vi "bitpacking_acquire_push.vi"(8 "sample":i16, 9 "Debug":bool=TRUE, 10 "Input Valid":bool, 11 "FIFO Refs":T1={"FIFO 0"="Simulation FIFO 0", "FIFO 1"="Simulation FIFO 1", "FIFO 2"="Simulation FIFO 2", "FIFO 3"="Simulation FIFO 3", "FIFO 4"="Simulation FIFO 4", "FIFO 5"="Simulation FIFO 5"}) -> (3 "Ready for Input":bool)   [LabVIEW 2014]
uses:
  FPGA_Controls/Acquisition FIFOs Cluster.ctl
  <vilib>/rvi/eio/common/nirviEmuTemplateMethod_errors.vi
  <vilib>/rvi/DataTransferAndStorage/Container/Common/niFpgaContainerExecOnDevCompGetState.vi
  <vilib>/rvi/Emulation/niFpgaEmulationIsFPGAContextNoSignature.vi
  <vilib>/rvi/Emulation/niFpgaSctlEmulationGetInTimedLoop.vi
  <vilib>/rvi/errors/niFpgaSetErrorForExecOnDevCompSimple.vi
  <vilib>/rvi/eio/common/nirviEmuReportErrorAndStop.vi
  <vilib>/rvi/DataTransferAndStorage/Container/Common/niFpgaContainerGetUniqueNameForEmu.vi
  <vilib>/rvi/FIFO/Fifo_Resource/nirvififoEmulationSetSize.vi
  <vilib>/rvi/FIFO/Fifo_Resource/nirviFifoEmulationQueueMgr.vi
  <instcachedir>/0/nirviFifoEmulationQueueMgr_E5CAEC123FF24DC58D834DCA3CDAA9B5.lvgen/nirviFifoEmulationQueueMgr_E5CAEC123FF24DC58D834DCA3CDAA9B5_003.vi
  <vilib>/rvi/FIFO/Fifo_Resource/nirvififoEmulationDetermineInputValidOut.vi
  <vilib>/rvi/FIFO/Fifo_Resource/nirvififoEmulationCreateLock.vi
  <vilib>/rvi/Emulation/niFpgaProcessEmulError.vi
  <vilib>/rvi/FIFO/Fifo_Resource/nirvififoEmulationObtainLock.vi
  <vilib>/rvi/FIFO/Fifo_Resource/nirvififoEmulationReleaseLock.vi
  <vilib>/rvi/occurrence/nirviWaitOnOccurrenceBase.vi
  <vilib>/rvi/errors/nirviReportUnexpectedCaseInternalError.vi
  <vilib>/rvi/errors/nirviReportUnexpectedCaseInternalError (U32).vi
  <vilib>/Utility/error.llb/Clear Errors.vi
  <vilib>/rvi/interface/RandomDataEmulation/niFpgaRandomDataHandleErrors.vi
  <vilib>/eio/EIONode/EIONode.xnode
  <vilib>/rvi/DataTransferAndStorage/Container/XNode/niFpgaContainer.xnode
  <vilib>/rvi/FIFO/Fifo_Resource/niFpgaFifoEmulationRefIn.vi
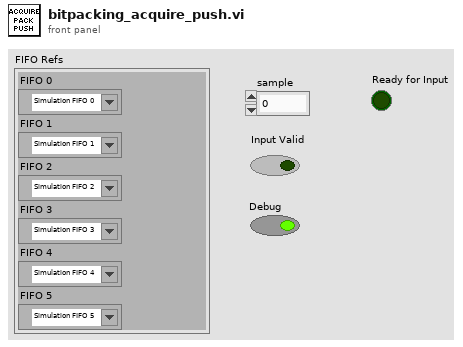
[diagram p1: front panel]
types:
  T1 = typedef "Acquisition FIFOs Cluster.ctl" = cluster{"FIFO 0":refnum<k21>, "FIFO 1":refnum<k21>, "FIFO 2":refnum<k21>, "FIFO 3":refnum<k21>, "FIFO 4":refnum<k21>, "FIFO 5":refnum<k21>}
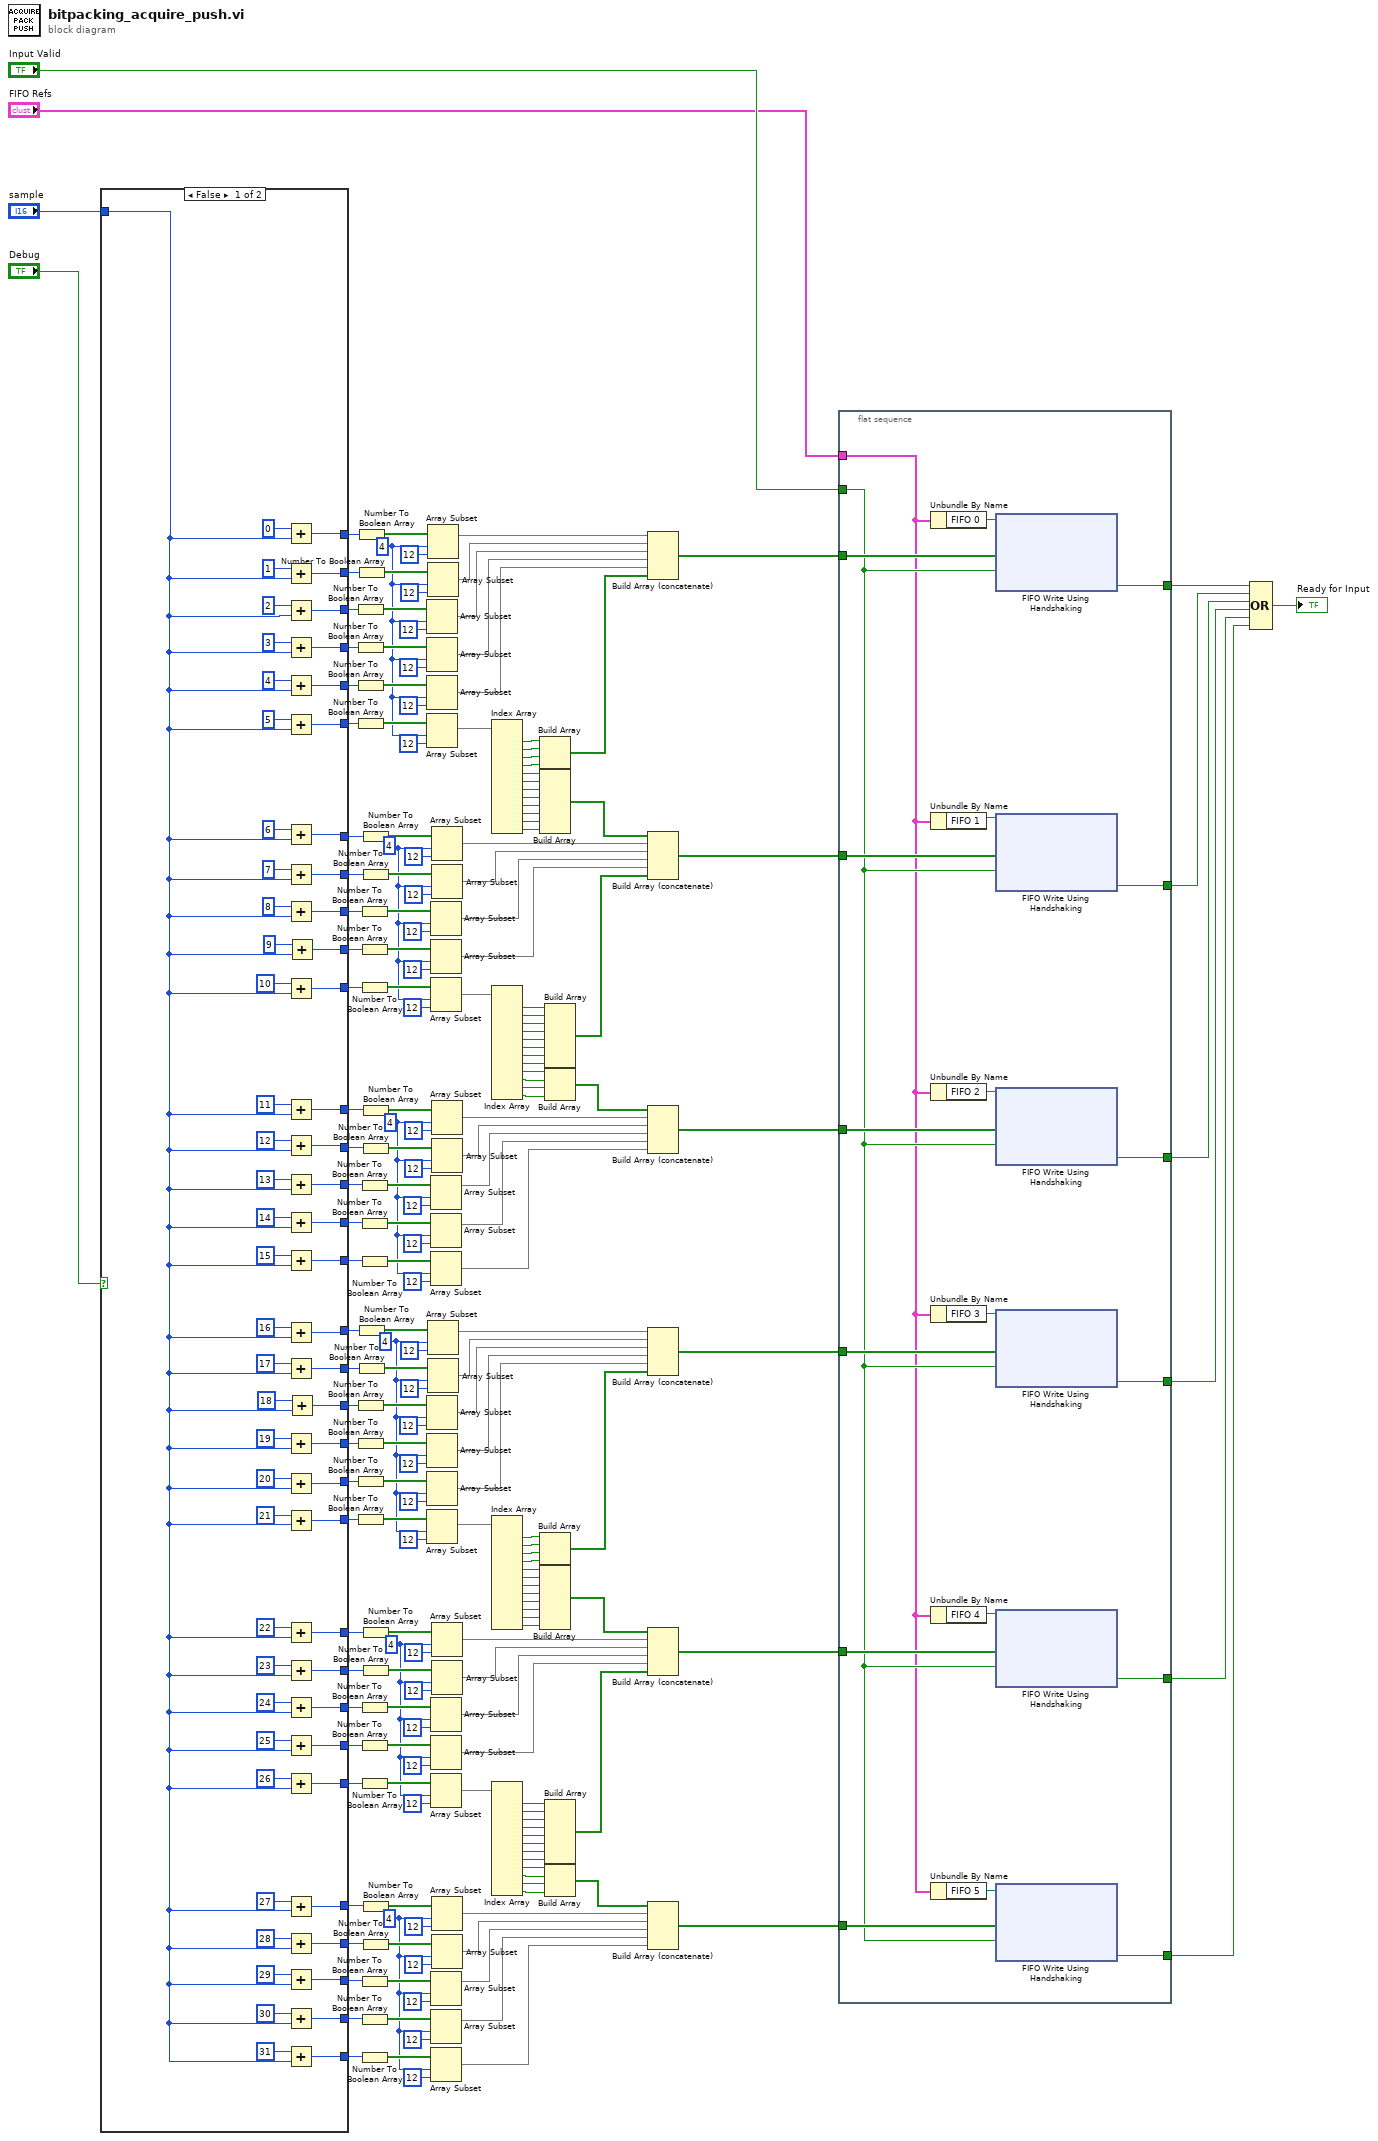
[diagram p0: block diagram]
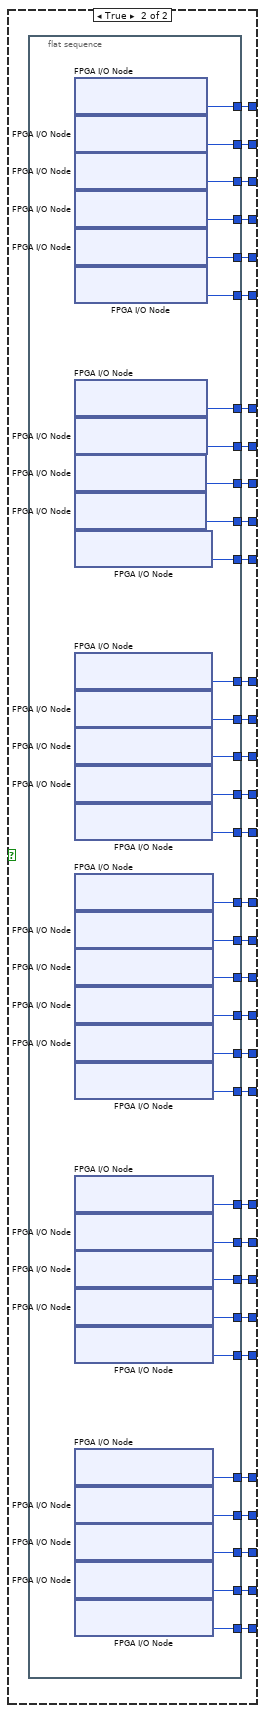
[diagram p2: hidden frame]
diagram:
  w3 = 4 ("length")
  w4 = 4 ("index")
  w5 = 4 ("index")
  w6 = 4 ("index")
  w7 = 4 ("index")
  w8 = 4 ("index")
  n1 = case shown="False" "Debug" {
    tunnel: [w219 w304] -> w125
    tunnel: [w218 w303] -> w124
    tunnel: [w217 w302] -> w123
    tunnel: [w216 w301] -> w122
    tunnel: [w215 w300] -> w121
    tunnel: [w214 w299] -> w120
    tunnel: [w213 w298] -> w119
    tunnel: [w212 w297] -> w118
    tunnel: [w211 w296] -> w117
    tunnel: [w210 w295] -> w116
    tunnel: [w209 w294] -> w115
    tunnel: [w240 w293] -> w114
    tunnel: [w239 w292] -> w113
    tunnel: [w238 w291] -> w112
    tunnel: [w237 w290] -> w111
    tunnel: [w236 w289] -> w110
    tunnel: [w220 w288] -> w103
    tunnel: [w221 w287] -> w102
    tunnel: [w222 w286] -> w101
    tunnel: [w223 w285] -> w100
    tunnel: [w224 w284] -> w99
    tunnel: [w225 w283] -> w98
    tunnel: [w226 w282] -> w97
    tunnel: [w227 w281] -> w96
    tunnel: [w228 w280] -> w95
    tunnel: [w229 w279] -> w94
    tunnel: [w230 w278] -> w93
    tunnel: [w231 w277] -> w92
    tunnel: [w232 w276] -> w91
    tunnel: [w233 w275] -> w90
    tunnel: [w234 w274] -> w89
    tunnel: [w235 w273] -> w88
    tunnel: "sample" -> [w208 _]
    frame False {
      n2 = Add(x=i16 0, y=w208) -> (x+y=w235:i16)
      n3 = Add(x=i16 1, y=w208) -> (x+y=w234:i16)
      n4 = Add(x=i16 2, y=w208) -> (x+y=w233:i16)
      n5 = Add(x=i16 3, y=w208) -> (x+y=w232:i16)
      n6 = Add(x=i16 4, y=w208) -> (x+y=w231:i16)
      n7 = Add(x=i16 5, y=w208) -> (x+y=w230:i16)
      n8 = Add(x=i16 6, y=w208) -> (x+y=w229:i16)
      n9 = Add(x=i16 7, y=w208) -> (x+y=w228:i16)
      n10 = Add(x=i16 8, y=w208) -> (x+y=w227:i16)
      n11 = Add(x=i16 10, y=w208) -> (x+y=w225:i16)
      n12 = Add(x=i16 11, y=w208) -> (x+y=w224:i16)
      n13 = Add(x=i16 12, y=w208) -> (x+y=w223:i16)
      n14 = Add(x=i16 13, y=w208) -> (x+y=w222:i16)
      n15 = Add(x=i16 14, y=w208) -> (x+y=w221:i16)
      n16 = Add(x=i16 15, y=w208) -> (x+y=w220:i16)
      n17 = Add(x=i16 16, y=w208) -> (x+y=w219:i16)
      n18 = Add(x=i16 17, y=w208) -> (x+y=w218:i16)
      n19 = Add(x=i16 19, y=w208) -> (x+y=w216:i16)
      n20 = Add(x=i16 20, y=w208) -> (x+y=w215:i16)
      n21 = Add(x=i16 21, y=w208) -> (x+y=w214:i16)
      n22 = Add(x=i16 22, y=w208) -> (x+y=w213:i16)
      n23 = Add(x=i16 23, y=w208) -> (x+y=w212:i16)
      n24 = Add(x=i16 24, y=w208) -> (x+y=w211:i16)
      n25 = Add(x=i16 25, y=w208) -> (x+y=w210:i16)
      n26 = Add(x=i16 26, y=w208) -> (x+y=w209:i16)
      n27 = Add(x=i16 27, y=w208) -> (x+y=w240:i16)
      n28 = Add(x=i16 28, y=w208) -> (x+y=w239:i16)
      n29 = Add(x=i16 29, y=w208) -> (x+y=w238:i16)
      n30 = Add(x=i16 30, y=w208) -> (x+y=w237:i16)
      n31 = Add(x=i16 31, y=w208) -> (x+y=w236:i16)
      n32 = Add(x=i16 9, y=w208) -> (x+y=w226:i16)
      n33 = Add(x=i16 18, y=w208) -> (x+y=w217:i16)
    }
    frame True {
      n34 = flat-sequence {
        tunnel: [w336] -> w273
        tunnel: [w335] -> w274
        tunnel: [w334] -> w275
        tunnel: [w333] -> w276
        tunnel: [w332] -> w277
        tunnel: [w331] -> w278
        tunnel: [w330] -> w279
        tunnel: [w329] -> w280
        tunnel: [w328] -> w281
        tunnel: [w327] -> w282
        tunnel: [w326] -> w283
        tunnel: [w325] -> w284
        tunnel: [w324] -> w285
        tunnel: [w323] -> w286
        tunnel: [w322] -> w287
        tunnel: [w321] -> w288
        tunnel: [w320] -> w289
        tunnel: [w319] -> w290
        tunnel: [w318] -> w291
        tunnel: [w317] -> w292
        tunnel: [w316] -> w293
        tunnel: [w315] -> w294
        tunnel: [w314] -> w295
        tunnel: [w313] -> w296
        tunnel: [w312] -> w297
        tunnel: [w311] -> w298
        tunnel: [w310] -> w299
        tunnel: [w309] -> w300
        tunnel: [w308] -> w301
        tunnel: [w307] -> w302
        tunnel: [w306] -> w303
        tunnel: [w305] -> w304
        frame #0 {
          n35 = xnode "FPGA I/O Node"() -> ("IO Module\\AI A0"=w336:i16)  [unwired: 1 in, 1 out]
          n36 = xnode "FPGA I/O Node"() -> ("IO Module\\AI A1"=w335:i16)  [unwired: 1 in, 1 out]
          n37 = xnode "FPGA I/O Node"() -> ("IO Module\\AI A2"=w334:i16)  [unwired: 1 in, 1 out]
          n38 = xnode "FPGA I/O Node"() -> ("IO Module\\AI A3"=w333:i16)  [unwired: 1 in, 1 out]
          n39 = xnode "FPGA I/O Node"() -> ("IO Module\\AI A4"=w332:i16)  [unwired: 1 in, 1 out]
          n40 = xnode "FPGA I/O Node"() -> ("IO Module\\AI A5"=w331:i16)  [unwired: 1 in, 1 out]
          n41 = xnode "FPGA I/O Node"() -> ("IO Module\\AI A6"=w330:i16)  [unwired: 1 in, 1 out]
          n42 = xnode "FPGA I/O Node"() -> ("IO Module\\AI A7"=w329:i16)  [unwired: 1 in, 1 out]
          n43 = xnode "FPGA I/O Node"() -> ("IO Module\\AI B8"=w328:i16)  [unwired: 1 in, 1 out]
          n44 = xnode "FPGA I/O Node"() -> ("IO Module\\AI B9"=w327:i16)  [unwired: 1 in, 1 out]
          n45 = xnode "FPGA I/O Node"() -> ("IO Module\\AI B10"=w326:i16)  [unwired: 1 in, 1 out]
          n46 = xnode "FPGA I/O Node"() -> ("IO Module\\AI B11"=w325:i16)  [unwired: 1 in, 1 out]
          n47 = xnode "FPGA I/O Node"() -> ("IO Module\\AI B12"=w324:i16)  [unwired: 1 in, 1 out]
          n48 = xnode "FPGA I/O Node"() -> ("IO Module\\AI B13"=w323:i16)  [unwired: 1 in, 1 out]
          n49 = xnode "FPGA I/O Node"() -> ("IO Module\\AI B14"=w322:i16)  [unwired: 1 in, 1 out]
          n50 = xnode "FPGA I/O Node"() -> ("IO Module\\AI B15"=w321:i16)  [unwired: 1 in, 1 out]
          n51 = xnode "FPGA I/O Node"() -> ("IO Module\\AI C16"=w305:i16)  [unwired: 1 in, 1 out]
          n52 = xnode "FPGA I/O Node"() -> ("IO Module\\AI C17"=w306:i16)  [unwired: 1 in, 1 out]
          n53 = xnode "FPGA I/O Node"() -> ("IO Module\\AI C18"=w307:i16)  [unwired: 1 in, 1 out]
          n54 = xnode "FPGA I/O Node"() -> ("IO Module\\AI C19"=w308:i16)  [unwired: 1 in, 1 out]
          n55 = xnode "FPGA I/O Node"() -> ("IO Module\\AI C20"=w309:i16)  [unwired: 1 in, 1 out]
          n56 = xnode "FPGA I/O Node"() -> ("IO Module\\AI C21"=w310:i16)  [unwired: 1 in, 1 out]
          n57 = xnode "FPGA I/O Node"() -> ("IO Module\\AI C22"=w311:i16)  [unwired: 1 in, 1 out]
          n58 = xnode "FPGA I/O Node"() -> ("IO Module\\AI C23"=w312:i16)  [unwired: 1 in, 1 out]
          n59 = xnode "FPGA I/O Node"() -> ("IO Module\\AI D24"=w313:i16)  [unwired: 1 in, 1 out]
          n60 = xnode "FPGA I/O Node"() -> ("IO Module\\AI D25"=w314:i16)  [unwired: 1 in, 1 out]
          n61 = xnode "FPGA I/O Node"() -> ("IO Module\\AI D26"=w315:i16)  [unwired: 1 in, 1 out]
          n62 = xnode "FPGA I/O Node"() -> ("IO Module\\AI D27"=w316:i16)  [unwired: 1 in, 1 out]
          n63 = xnode "FPGA I/O Node"() -> ("IO Module\\AI D28"=w317:i16)  [unwired: 1 in, 1 out]
          n64 = xnode "FPGA I/O Node"() -> ("IO Module\\AI D29"=w318:i16)  [unwired: 1 in, 1 out]
          n65 = xnode "FPGA I/O Node"() -> ("IO Module\\AI D30"=w319:i16)  [unwired: 1 in, 1 out]
          n66 = xnode "FPGA I/O Node"() -> ("IO Module\\AI D31"=w320:i16)  [unwired: 1 in, 1 out]
        }
      }
    }
  }
  n67 = Number To Boolean Array(number=w90) -> (Boolean array=w21:bool[])
  n68 = Number To Boolean Array(number=w91) -> (Boolean array=w18:bool[])
  n69 = Number To Boolean Array(number=w92) -> (Boolean array=w27:bool[])
  n70 = Number To Boolean Array(number=w93) -> (Boolean array=w24:bool[])
  n71 = Number To Boolean Array(number=w123) -> (Boolean array=w192:bool[])
  n72 = Number To Boolean Array(number=w122) -> (Boolean array=w195:bool[])
  n73 = Number To Boolean Array(number=w121) -> (Boolean array=w186:bool[])
  n74 = Number To Boolean Array(number=w120) -> (Boolean array=w189:bool[])
  n75 = Number To Boolean Array(number=w88) -> (Boolean array=w12:bool[])
  n76 = Number To Boolean Array(number=w89) -> (Boolean array=w15:bool[])
  n77 = Number To Boolean Array(number=w125) -> (Boolean array=w201:bool[])
  n78 = Number To Boolean Array(number=w124) -> (Boolean array=w198:bool[])
  n79 = Number To Boolean Array(number=w96) -> (Boolean array=w45:bool[])
  n80 = Number To Boolean Array(number=w97) -> (Boolean array=w48:bool[])
  n81 = Number To Boolean Array(number=w98) -> (Boolean array=w43:bool[])
  n82 = Number To Boolean Array(number=w101) -> (Boolean array=w79:bool[])
  n83 = Number To Boolean Array(number=w102) -> (Boolean array=w76:bool[])
  n84 = Number To Boolean Array(number=w103) -> (Boolean array=w81:bool[])
  n85 = Number To Boolean Array(number=w117) -> (Boolean array=w168:bool[])
  n86 = Number To Boolean Array(number=w116) -> (Boolean array=w165:bool[])
  n87 = Number To Boolean Array(number=w115) -> (Boolean array=w170:bool[])
  n88 = Number To Boolean Array(number=w112) -> (Boolean array=w134:bool[])
  n89 = Number To Boolean Array(number=w111) -> (Boolean array=w137:bool[])
  n90 = Number To Boolean Array(number=w110) -> (Boolean array=w132:bool[])
  n91 = Number To Boolean Array(number=w94) -> (Boolean array=w52:bool[])
  n92 = Number To Boolean Array(number=w95) -> (Boolean array=w49:bool[])
  n93 = Number To Boolean Array(number=w99) -> (Boolean array=w72:bool[])
  n94 = Number To Boolean Array(number=w100) -> (Boolean array=w75:bool[])
  n95 = Number To Boolean Array(number=w119) -> (Boolean array=w161:bool[])
  n96 = Number To Boolean Array(number=w118) -> (Boolean array=w164:bool[])
  n97 = Number To Boolean Array(number=w114) -> (Boolean array=w141:bool[])
  n98 = Number To Boolean Array(number=w113) -> (Boolean array=w138:bool[])
  n99 = Array Subset(array=w21, index=w8, length=12) -> (w22:bool[])
  n100 = Array Subset(array=w18, index=w8, length=12) -> (w23:bool[])
  n101 = Array Subset(array=w27, index=w8, length=12) -> (w28:bool[])
  n102 = Array Subset(array=w24, index=w8, length=12) -> (w29:bool[])
  n103 = Array Subset(array=w192, index=w5, length=12) -> (w191:bool[])
  n104 = Array Subset(array=w195, index=w5, length=12) -> (w190:bool[])
  n105 = Array Subset(array=w186, index=w5, length=12) -> (w185:bool[])
  n106 = Array Subset(array=w189, index=w5, length=12) -> (w184:bool[])
  n107 = Array Subset(array=w12, index=w8, length=12) -> (w16:bool[])
  n108 = Array Subset(array=w15, index=w8, length=12) -> (w17:bool[])
  n109 = Array Subset(array=w201, index=w5, length=12) -> (w197:bool[])
  n110 = Array Subset(array=w198, index=w5, length=12) -> (w196:bool[])
  n111 = Array Subset(array=w45, index=w7, length=12) -> (w56:bool[])
  n112 = Array Subset(array=w48, index=w7, length=12) -> (w57:bool[])
  n113 = Array Subset(array=w43, index=w7, length=12) -> (w58:bool[])
  n114 = Array Subset(array=w79, index=w6, length=12) -> (w85:bool[])
  n115 = Array Subset(array=w76, index=w6, length=12) -> (w86:bool[])
  n116 = Array Subset(array=w81, index=w6, length=12) -> (w87:bool[])
  n117 = Array Subset(array=w168, index=w4, length=12) -> (w157:bool[])
  n118 = Array Subset(array=w165, index=w4, length=12) -> (w156:bool[])
  n119 = Array Subset(array=w170, index=w4, length=12) -> (w155:bool[])
  n120 = Array Subset(array=w134, index=w3, length=12) -> (w128:bool[])
  n121 = Array Subset(array=w137, index=w3, length=12) -> (w127:bool[])
  n122 = Array Subset(array=w132, index=w3, length=12) -> (w126:bool[])
  n123 = Array Subset(array=w52, index=w7, length=12) -> (w54:bool[])
  n124 = Array Subset(array=w49, index=w7, length=12) -> (w55:bool[])
  n125 = Array Subset(array=w72, index=w6, length=12) -> (w83:bool[])
  n126 = Array Subset(array=w75, index=w6, length=12) -> (w84:bool[])
  n127 = Array Subset(array=w161, index=w4, length=12) -> (w159:bool[])
  n128 = Array Subset(array=w164, index=w4, length=12) -> (w158:bool[])
  n129 = Array Subset(array=w141, index=w3, length=12) -> (w130:bool[])
  n130 = Array Subset(array=w138, index=w3, length=12) -> (w129:bool[])
  n131 = Index Array(array=w29) -> (element #1=w30:bool, element #2=w31:bool, element #3=w32:bool, element #4=w33:bool, element #5=w35:bool, element #6=w36:bool, element #7=w37:bool, element #8=w38:bool, element #9=w39:bool, element #10=w40:bool, element #11=w41:bool, element #12=w42:bool)  [unwired: 12 in]
  n132 = Index Array(array=w58) -> (element #1=w59:bool, element #2=w60:bool, element #3=w61:bool, element #4=w62:bool, element #5=w63:bool, element #6=w64:bool, element #7=w65:bool, element #8=w66:bool, element #9=w68:bool, element #10=w69:bool, element #11=w70:bool, element #12=w71:bool)  [unwired: 12 in]
  n133 = Index Array(array=w184) -> (element #1=w183:bool, element #2=w182:bool, element #3=w181:bool, element #4=w180:bool, element #5=w178:bool, element #6=w177:bool, element #7=w176:bool, element #8=w175:bool, element #9=w174:bool, element #10=w173:bool, element #11=w172:bool, element #12=w171:bool)  [unwired: 12 in]
  n134 = Index Array(array=w155) -> (element #1=w154:bool, element #2=w153:bool, element #3=w152:bool, element #4=w151:bool, element #5=w150:bool, element #6=w149:bool, element #7=w148:bool, element #8=w147:bool, element #9=w145:bool, element #10=w144:bool, element #11=w143:bool, element #12=w142:bool)  [unwired: 12 in]
  n135 = Build Array(w30, w31, w32, w33) -> (w34:bool[])
  n136 = Build Array(w35, w36, w37, w38, w39, w40, w41, w42) -> (w53:bool[])
  n137 = Build Array(w183, w182, w181, w180) -> (w179:bool[])
  n138 = Build Array(w178, w177, w176, w175, w174, w173, w172, w171) -> (w160:bool[])
  n139 = Build Array(w59, w60, w61, w62, w63, w64, w65, w66) -> (w67:bool[])
  n140 = Build Array(w68, w69, w70, w71) -> (w82:bool[])
  n141 = Build Array(w154, w153, w152, w151, w150, w149, w148, w147) -> (w146:bool[])
  n142 = Build Array(w145, w144, w143, w142) -> (w131:bool[])
  n143 = Build Array (concatenate)(w16, w17, w22, w23, w28, w34) -> (w104:bool[])
  n144 = Build Array (concatenate)(w53, w54, w55, w56, w57, w67) -> (w105:bool[])
  n145 = Build Array (concatenate)(w82, w83, w84, w85, w86, w87) -> (w106:bool[])
  n146 = Build Array (concatenate)(w197, w196, w191, w190, w185, w179) -> (w109:bool[])
  n147 = Build Array (concatenate)(w160, w159, w158, w157, w156, w146) -> (w108:bool[])
  n148 = Build Array (concatenate)(w131, w130, w129, w128, w127, w126) -> (w107:bool[])
  n149 = flat-sequence {
    tunnel: w104 -> [w356]
    tunnel: w105 -> [w355]
    tunnel: w106 -> [w354]
    tunnel: w107 -> [w353]
    tunnel: w108 -> [w352]
    tunnel: w109 -> [w351]
    tunnel: [w350] -> w202
    tunnel: [w349] -> w203
    tunnel: [w348] -> w204
    tunnel: [w347] -> w205
    tunnel: [w346] -> w206
    tunnel: [w345] -> w207
    tunnel: "Input Valid" -> [w344]
    tunnel: "FIFO Refs" -> [w337]
    frame #0 {
      n150 = Unbundle By Name(w337) -> ("FIFO 0"=w343:refnum<k21>)
      n151 = Unbundle By Name(w337) -> ("FIFO 1"=w342:refnum<k21>)
      n152 = Unbundle By Name(w337) -> ("FIFO 2"=w341:refnum<k21>)
      n153 = Unbundle By Name(w337) -> ("FIFO 3"=w340:refnum<k21>)
      n154 = Unbundle By Name(w337) -> ("FIFO 4"=w339:refnum<k21>)
      n155 = Unbundle By Name(w337) -> ("FIFO 5"=w338:refnum<k21>)
      n156 = xnode ("FIFO Write Using Handshaking")("Element"=w356, "Input Valid"=w344, "FIFO In"=w343) -> ("Ready for Input"=w350:bool)  [unwired: 1 out]
      n157 = xnode ("FIFO Write Using Handshaking")("Element"=w355, "Input Valid"=w344, "FIFO In"=w342) -> ("Ready for Input"=w349:bool)  [unwired: 1 out]
      n158 = xnode ("FIFO Write Using Handshaking")("Element"=w354, "Input Valid"=w344, "FIFO In"=w341) -> ("Ready for Input"=w348:bool)  [unwired: 1 out]
      n159 = xnode ("FIFO Write Using Handshaking")("Element"=w351, "Input Valid"=w344, "FIFO In"=w340) -> ("Ready for Input"=w347:bool)  [unwired: 1 out]
      n160 = xnode ("FIFO Write Using Handshaking")("Element"=w352, "Input Valid"=w344, "FIFO In"=w339) -> ("Ready for Input"=w346:bool)  [unwired: 1 out]
      n161 = xnode ("FIFO Write Using Handshaking")("Element"=w353, "Input Valid"=w344, "FIFO In"=w338) -> ("Ready for Input"=w345:bool)  [unwired: 1 out]
    }
  }
  n162 = Compound Arithmetic op=OR(w202, w203, w204, w205, w206, w207) -> (→"Ready for Input":bool)
